vi "Read TraceMessage.vi"(8 "error in (no error)":errorcluster, 11 "Tracer in":refnum<class "Tracer.lvclass">) -> (0 "error out":errorcluster, 2 "TraceMessage.lvclass":refnum<class "Trace.lvclass">, 3 "Tracer out":refnum<class "Tracer.lvclass">)   [LabVIEW 2013, in "Tracer.lvclass"]
uses:
  Tracer.lvclass
  TraceMessage/Trace.lvclass
  Tracer.lvclass/Tracer.ctl
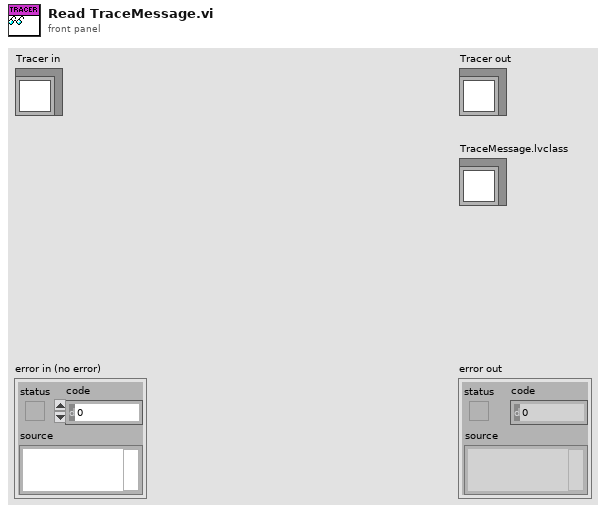
[diagram p1: front panel]
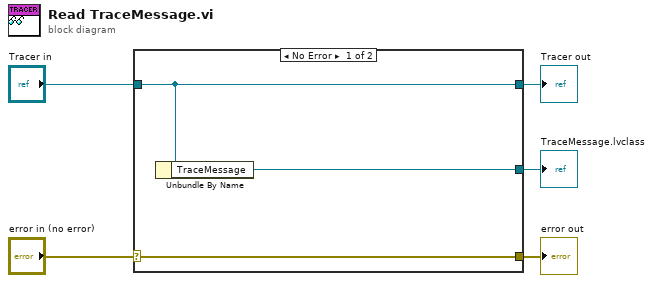
[diagram p0: block diagram]
diagram:
  n1 = case shown="No Error" "error in (no error)" {
    selector: "error in (no error)" -> [w8 w9]
    tunnel: [w8 w9] -> w4
    tunnel: [w7 w10] -> w2
    tunnel: "Tracer in" -> [w7 w10]
    tunnel: [w6 _] -> w1
    frame No Error {
      n2 = Unbundle By Name(w7) -> ("TraceMessage"=w6:refnum<class "Trace.lvclass">)
    }
    frame Error {
    }
  }
  "error out" <- w4
  "Tracer out" <- w2
  "TraceMessage.lvclass" <- w1
